vi "Generate And Open PFD.vi"(8 "error in":errorcluster, 10 "Generated File Path":path, 11 "Open Generated Document":bool=TRUE) -> (0 "error out":errorcluster)   [LabVIEW 2020, in "Panther Dashboard.lvlib"]
uses:
  Panther Dashboard.lvlib
  <vilib>/Wovalab/AsciiDoc for LabVIEW/Toolchain/Output Format--enum.ctl
  <vilib>/Wovalab/AsciiDoc for LabVIEW/Wovalab_lib_AsciiDoctor.lvlib
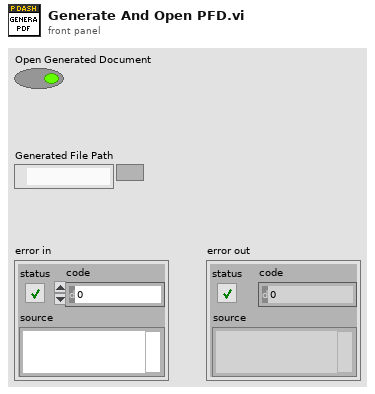
[diagram p1: front panel]
types:
  T1 = typedef "Wovalab_lib_AsciiDoctor.lvlib/Output Format--enum.ctl" = enum16{"HTML5", "PDF"}
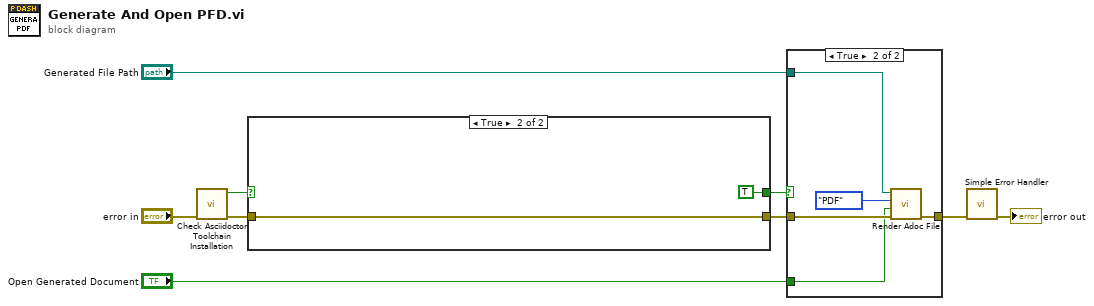
[diagram p0: block diagram]
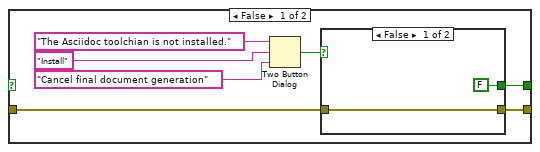
[diagram p3: hidden frame]
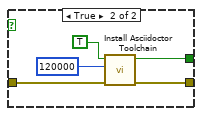
[diagram p4: hidden frame]
diagram:
  n1 = call <vilib>:"Check Asciidoctor Toolchain Installation.vi"("error in"="error in") -> ("error out"=w8:errorcluster, "Installation Ok?"=w3:bool)  [unwired: 8 in, 1 out]
  n2 = case shown="True" w3 {
    tunnel: w8 -> [w16 w25]
    tunnel: [w15 w25] -> w7
    tunnel: [w10 TRUE ("Successfull?")] -> w2
    frame False {
      n3 = Two Button Dialog(message="The Asciidoc toolchian is not installed.", 1:"Cancel final document generation" ("F button name (\"Cancel\")"), 2:"Install" ("T button name (\"OK\")")) -> (T button?=w11:bool)
      n4 = case shown="False" w11 {
        tunnel: w16 -> [w18 w23]
        tunnel: [w18 w22] -> w15
        tunnel: [FALSE ("Successfull?") w19] -> w10
        frame False {
        }
        frame True {
          n5 = call <vilib>:"Install Asciidoctor Toolchain.vi"("error in"=w23, "Dowload Timeout (60000ms)"=u32 120000, "Verbose"=TRUE) -> ("error out"=w22:errorcluster, "Successfull?"=w19:bool)  [unwired: 6 in, 1 out]
        }
      }
    }
    frame True {
    }
  }
  n6 = case shown="True" w2 {
    tunnel: [w26 w31] -> w5
    tunnel: "Generated File Path" -> [_ w29]
    tunnel: w7 -> [w26 w30]
    tunnel: "Open Generated Document" -> [_ w28]
    frame False {
    }
    frame True {
      n7 = call <vilib>:"Render Adoc File.vi"("error in"=w30, "Open Generated Document"=w28, "Output Format"=Output_Format--enum."PDF", "Adoc File Path"=w29) -> ("error out"=w31:errorcluster)  [unwired: 4 in, 3 out]
    }
  }
  n8 = call <vilib>:"Simple Error Handler.vi"("error in (no error)"=w5) -> ("error out"=→"error out":errorcluster)  [unwired: 4 in, 4 out]
